vi "Init.vi"(8 "error in (no error)":errorcluster, 11 "CameraTestingUI in":refnum<class "CameraTestingUI.lvclass">) -> (0 "error out":errorcluster, 3 "CameraTestingUI out":refnum<class "CameraTestingUI.lvclass">)   [LabVIEW 2020, in "CameraTestingUI.lvlib" / "CameraTestingUI.lvclass"]
uses:
  CameraTestingUI.lvclass
  C:/Program Files (x86)/National Instruments/LabVIEW 2020/vi.lib/ActorFramework/Actor/Actor.lvclass
  Private/TypeDef/ConnectionStatus.ctl
  CameraTestingUI.lvclass/CameraTestingUI.ctl
  <vilib>/ActorFramework/Actor/Actor.lvclass/Actor.ctl
  <vilib>/ActorFramework/Message Enqueuer/Message Enqueuer.lvclass/Message Enqueuer.ctl
  ICameraTesting/ICameraTesting Messages/LoadIntoSubPanel Msg/LoadIntoSubPanel Msg.lvclass/LoadIntoSubPanel Msg.ctl
  <vilib>/ActorFramework/Message Enqueuer/Enqueue.vi
  ICameraTesting/ICameraTesting Messages/AcqVideoOptCodes Msg/AcqVideoOptCodes Msg.lvclass
  C:/Program Files (x86)/National Instruments/LabVIEW 2020/vi.lib/ActorFramework/Message/Message.lvclass
  ICameraTesting/ICameraTesting Messages/LoadIntoSubPanel Msg/LoadIntoSubPanel Msg.lvclass
  <vilib>/ActorFramework/Message Priority Queue/Priority Enqueue.vi
  <vilib>/ActorFramework/Actor/Actor.lvclass
  ICameraTesting/ICameraTesting Messages/GetEvents Msg/GetEvents Msg.lvclass
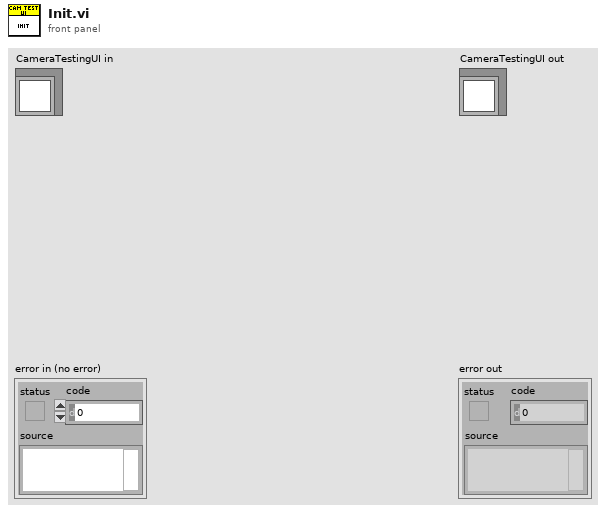
[diagram p1: front panel]
types:
  T1 = enum16{"Reset FP", "Get CameraTersting Events", "Request Video Options Values", "Open FP"}[]
  T2 = enum8{"Enabled", "Disabled", "Disabled and Grayed Out"}
  T3 = typedef "CameraTestingUI.lvlib/CameraTestingUI.lvclass/ConnectionStatus.ctl" = u16
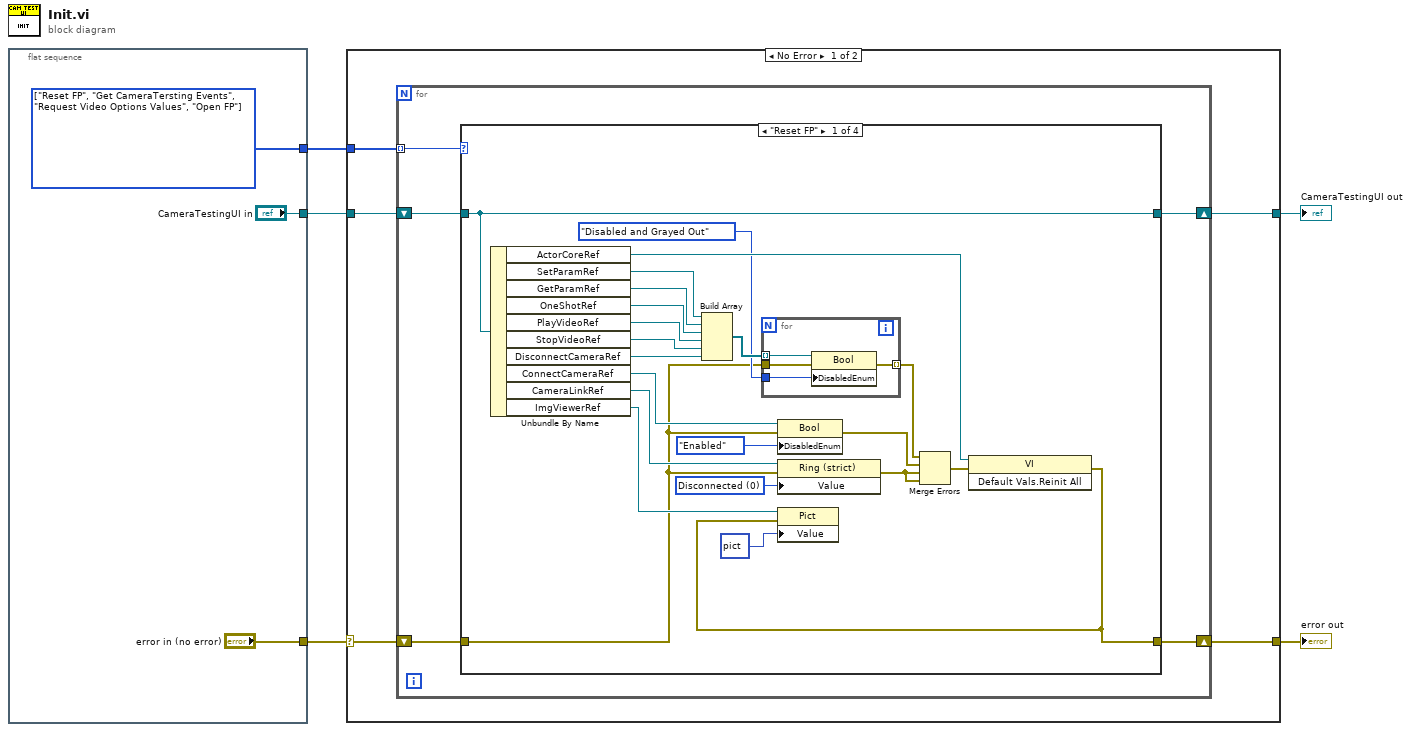
[diagram p0: block diagram]
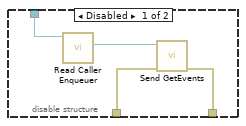
[diagram p3: hidden frame]
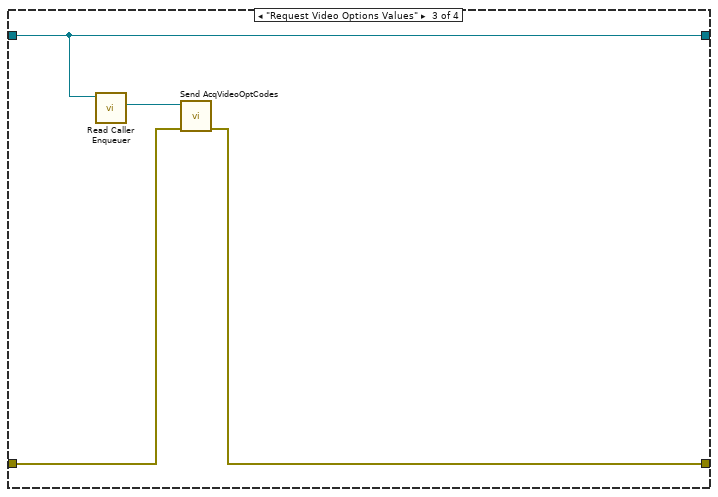
[diagram p4: hidden frame]
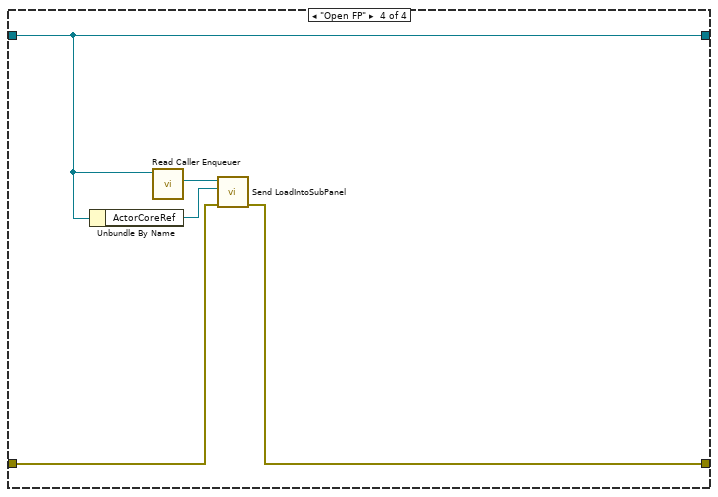
[diagram p5: hidden frame]
diagram:
  n1 = flat-sequence {
    tunnel: ["error in (no error)"] -> w5
    tunnel: ["CameraTestingUI in"] -> w3
    tunnel: [w6] -> w1
    frame #0 {
      w6 = T1 [enum."Reset FP", enum."Get CameraTersting Events", enum."Request Video Options Values", enum."Open FP"] items=["Reset FP", "Get CameraTersting Events", "Request Video Options Values", "Open FP"]
    }
  }
  n2 = case shown="No Error" w5 {
    selector: w5 -> [w12 w63]
    tunnel: [w11 w63] -> w4
    tunnel: [w10 w62] -> w2
    tunnel: w3 -> [w13 w62]
    tunnel: w1 -> [w9 _]
    frame No Error {
      n3 = for {
        shift-right: [w15] -> w10
        shift-left: w13 -> [w16]
        shift-right: [w17] -> w11
        shift-left: w12 -> [w18]
        tunnel: w9 -> [w14] mode=indexing
        n4 = case shown="\"Reset FP\"" w14 {
          tunnel: w18 -> [w21 w46 w54 w61]
          tunnel: [w20 w45 w53 w60] -> w17
          tunnel: w16 -> [w40 w47 w56 w58]
          tunnel: [w40 w47 w56 w58] -> w15
          frame "Reset FP" {
            w24 = T3 0 items=["Disconnected", "Connected", "Error"] ("Value")
            n5 = Unbundle By Name(w40) -> ("ActorCoreRef"=w26:refnum<vi>, "SetParamRef"=w36:refnum<vi>, "GetParamRef"=w35:refnum<vi>, "OneShotRef"=w34:refnum<vi>, "PlayVideoRef"=w33:refnum<vi>, "StopVideoRef"=w32:refnum<vi>, "DisconnectCameraRef"=w31:refnum<vi>, "ConnectCameraRef"=w30:refnum<vi>, "CameraLinkRef"=w29:refnum<vi>, "ImgViewerRef"=w23:refnum<vi>)
            n6 = Build Array(w36, w35, w34, w33, w32, w31) -> (w39:refnum<vi>[])
            n7 = for {
              tunnel: w39 -> [w44] mode=indexing
              tunnel: w21 -> [w43]
              tunnel: [w42] -> w38 mode=indexing
              tunnel: T2."Disabled and Grayed Out" ("Disabled") -> [w41]
              n8 = property class="Bool"(reference=w44, error in=w43, "DisabledEnum"=w41) -> (error out=w42:errorcluster)  [unwired: 1 out]
            }
            n9 = property class="Bool"(reference=w30, error in=w21, "DisabledEnum"=T2."Enabled" ("Disabled")) -> (error out=w37:errorcluster)  [unwired: 1 out]
            n10 = property class="Ring (strict)"(reference=w29, error in=w21, "Value"=w24) -> (error out=w19:errorcluster)  [unwired: 1 out]
            n11 = Merge Errors(w38, w37, w19, w19) -> (w27:errorcluster)
            n12 = invoke class="VI" method="Default Vals.Reinit All"(reference=w26, error in=w27) -> (error out=w20:errorcluster)  [unwired: 1 in, 2 out]
            n13 = property class="Pict"(reference=w23, error in=w20, "Value"=picture data[5B]) -> ()  [unwired: 2 out]
          }
          frame "Get CameraTersting Events" {
            n14 = disable-structure shown="Enabled" {
              disable-tunnel: w47 -> [w51 _]
              disable-tunnel: w46 -> [w49 w52]
              disable-tunnel: [w48 w52] -> w45
              frame Disabled {
                n15 = call <vilib>:"Read Caller Enqueuer.vi"("Actor"=w51) -> ("Caller Enqueuer"=w50:refnum<class "Message Enqueuer.lvclass">)  [unwired: 10 in]
                n16 = call "Send GetEvents.vi"("error in (no error)"=w49, "Message Enqueuer"=w50) -> ("error out"=w48:errorcluster)  [unwired: 8 in, 1 out]
              }
              frame Enabled {
              }
            }
          }
          frame "Request Video Options Values" {
            n17 = call <vilib>:"Read Caller Enqueuer.vi"("Actor"=w56) -> ("Caller Enqueuer"=w55:refnum<class "Message Enqueuer.lvclass">)  [unwired: 10 in]
            n18 = call "Send AcqVideoOptCodes.vi"("error in (no error)"=w54, "Message Enqueuer"=w55) -> ("error out"=w53:errorcluster)  [unwired: 8 in, 1 out]
          }
          frame "Open FP" {
            n19 = Unbundle By Name(w58) -> ("ActorCoreRef"=w57:refnum<vi>)
            n20 = call <vilib>:"Read Caller Enqueuer.vi"("Actor"=w58) -> ("Caller Enqueuer"=w59:refnum<class "Message Enqueuer.lvclass">)  [unwired: 10 in]
            n21 = call "Send LoadIntoSubPanel.vi"("error in (no error)"=w61, "VI Refnum"=w57, "Message Enqueuer"=w59) -> ("error out"=w60:errorcluster)  [unwired: 7 in, 1 out]
          }
        }
      }
    }
    frame Error {
    }
  }
  "error out" <- w4
  "CameraTestingUI out" <- w2
